vi "create_default_fiile_diag.vi"() -> (0 "error out":errorcluster, 3 "Byte Stream File out":refnum<file>)   [LabVIEW 2015]
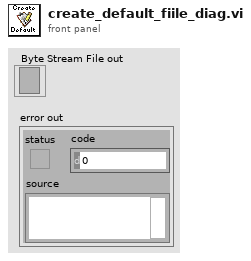
[diagram p1: front panel]
types:
  T1 = enum16{"open", "replace", "create", "open or create", "replace or create", "replace or create with confirmation"}
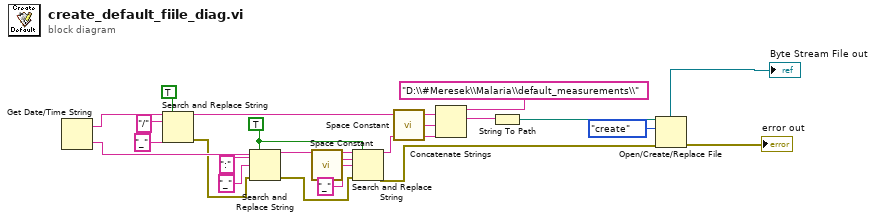
[diagram p0: block diagram]
diagram:
  w6 = TRUE ("replace all? (F)")
  n1 = Get Date/Time String() -> (date string=w9:string, time string=w19:string)  [unwired: 3 in]
  n2 = Search and Replace String(replace all?=TRUE ("replace all? (F)"), input string=w9, search string="/", replace string="_" ("replace string (\"\")")) -> (result string=w13:string, error out=w18:errorcluster)  [unwired: 4 in, 2 out]
  n3 = Search and Replace String(replace all?=w6, input string=w19, search string=":", replace string="_" ("replace string (\"\")"), error in=w18) -> (result string=w4:string, error out=w17:errorcluster)  [unwired: 3 in, 2 out]
  n4 = call <vilib>:"Space Constant.vi"() -> ("String"=w12:string)
  n5 = Search and Replace String(replace all?=w6, input string=w4, search string=w12, replace string="_" ("replace string (\"\")"), error in=w17) -> (result string=w14:string, error out=w20:errorcluster)  [unwired: 3 in, 2 out]
  n6 = call <vilib>:"Space Constant.vi"() -> ("String"=w15:string)
  n7 = Concatenate Strings("D:\\#Meresek\\Malaria\\default_measurements\\", w13, w15, w14) -> (w7:string)
  n8 = String To Path(string=w7) -> (path=w22:path)
  n9 = Open/Create/Replace File(file path (use dialog)=w22, error in=w20, operation (0:open)=T1."create") -> (refnum out=→"Byte Stream File out":refnum<file>, error out=→"error out":errorcluster)  [unwired: 3 in, 1 out]
